vi "Set Aout Limit.vi"(8 "error in (no error)":errorcluster, 9 "firmware revision":string(combo), 10 "aout limit":T2={"ALimUpC (10.5)"=10.5, "ALimUpL (10.5)"=10.0, "ALimLoC (-10.5)"=-10.0, "ALimLoL (-10.5)"=-10.0}, 11 "VISA resource name":refnum<visa-resource-name>) -> (0 "error out":errorcluster, 2 "bridge error":T1, 3 "VISA resource name out":refnum<visa-resource-name>)   [LabVIEW 2020, in "Andeen-Hagerling 2700A.lvlib"]
doc: "Sets the upper and lower protection limits, respectively, of\nthe capacitance and loss channel output voltages in volts.\nThese protection limits apply only to voltage levels produced\nby the deviation subsystem. They do not limit the output\nderived from internal bias voltage sources."
uses:
  Andeen-Hagerling 2700A.lvlib
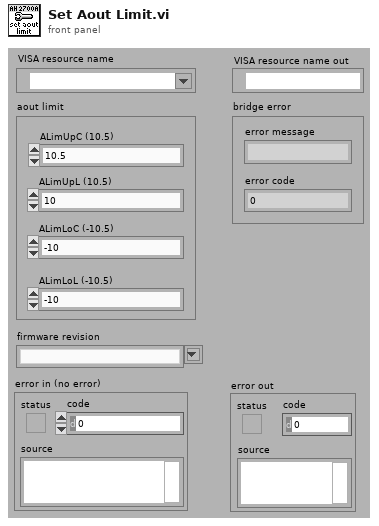
[diagram p1: front panel]
types:
  T1 = cluster{"error message":string, "error code":i32}
  T2 = cluster{"ALimUpC (10.5)":dbl, "ALimUpL (10.5)":dbl, "ALimLoC (-10.5)":dbl, "ALimLoL (-10.5)":dbl}
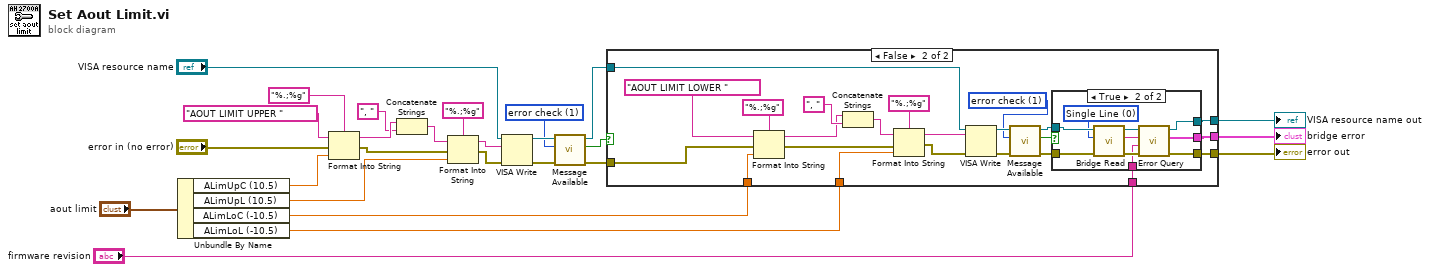
[diagram p0: block diagram]
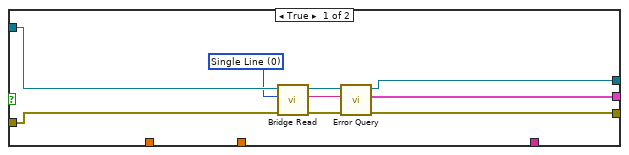
[diagram p2: hidden frame]
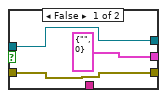
[diagram p3: hidden frame]
diagram:
  w1 = u16 1 items=["none", "error check", "multiline read", "infinite"] ("delay")
  n1 = Unbundle By Name("aout limit") -> ("ALimUpC (10.5)"=w17:dbl, "ALimUpL (10.5)"=w16:dbl, "ALimLoC (-10.5)"=w11:dbl, "ALimLoL (-10.5)"=w10:dbl)
  n2 = Format Into String(format string="%.;%g", initial string="AOUT LIMIT UPPER " ("command"), error in="error in (no error)", w17) -> (resulting string=w24:string, error out=w25:errorcluster)
  n3 = Concatenate Strings(w24, ", " ("command")) -> (w20:string)
  n4 = Format Into String(format string="%.;%g", initial string=w20, error in=w25, w16) -> (resulting string=w15:string, error out=w14:errorcluster)
  n5 = VISA Write(VISA resource name="VISA resource name", write buffer=w15, error in (no error)=w14) -> (VISA resource name out=w13:refnum<visa-resource-name>, error out=w12:errorcluster)  [unwired: 1 out]
  n6 = call "Message Available.vi"("error in (no error)"=w12, "delay"=w1, "VISA resource name"=w13) -> ("error out"=w3:errorcluster, "message available"=w2:bool, "VISA resource name out"=w4:refnum<visa-resource-name>)  [unwired: 6 in]
  n7 = case shown="False" w2 {
    tunnel: w11 -> [_ w44]
    tunnel: w10 -> [_ w43]
    tunnel: w4 -> [w31 w42]
    tunnel: "firmware revision" -> [_ w41]
    tunnel: [w30 w40] -> w8
    tunnel: [w29 w39] -> w7
    tunnel: [w28 w38] -> w6
    tunnel: w3 -> [w32 w37]
    frame True {
      w27 = u16 0 items=["Single Line", "Multi-Line"] ("Multiline")
      n8 = call "Bridge Read.vi"("error in (no error)"=w32, "multiline"=w27, "VISA resource name"=w31) -> ("error out"=w34:errorcluster, "read buffer"=w35:string, "VISA resource name out"=w33:refnum<visa-resource-name>)  [unwired: 6 in]
      n9 = call "Error Query.vi"("error in (no error)"=w34, "measurement line"=w35, "VISA resource name"=w33) -> ("error out"=w28:errorcluster, "bridge error"=w29:T1, "VISA resource name out"=w30:refnum<visa-resource-name>)  [unwired: 6 in]
    }
    frame False {
      w36 = u16 1 items=["none", "error check", "multiline read", "infinite"] ("delay")
      n10 = Format Into String(format string="%.;%g", initial string="AOUT LIMIT LOWER " ("command"), error in=w37, w44) -> (resulting string=w54:string, error out=w53:errorcluster)
      n11 = Concatenate Strings(w54, ", " ("command")) -> (w56:string)
      n12 = Format Into String(format string="%.;%g", initial string=w56, error in=w53, w43) -> (resulting string=w51:string, error out=w52:errorcluster)
      n13 = VISA Write(VISA resource name=w42, write buffer=w51, error in (no error)=w52) -> (VISA resource name out=w47:refnum<visa-resource-name>, error out=w46:errorcluster)  [unwired: 1 out]
      n14 = call "Message Available.vi"("error in (no error)"=w46, "delay"=w36, "VISA resource name"=w47) -> ("error out"=w48:errorcluster, "message available"=w50:bool, "VISA resource name out"=w49:refnum<visa-resource-name>)  [unwired: 6 in]
      n15 = case shown="True" w50 {
        tunnel: w49 -> [w60 w68]
        tunnel: w48 -> [w61 w67]
        tunnel: w41 -> [_ w66]
        tunnel: [w61 w65] -> w38
        tunnel: [w60 w64] -> w40
        tunnel: [T1 {"error message"="", "error code"=0} ("bridge error") w63] -> w39
        frame False {
        }
        frame True {
          w62 = u16 0 items=["Single Line", "Multi-Line"] ("Multiline")
          n16 = call "Bridge Read.vi"("error in (no error)"=w67, "multiline"=w62, "VISA resource name"=w68) -> ("error out"=w70:errorcluster, "read buffer"=w71:string, "VISA resource name out"=w69:refnum<visa-resource-name>)  [unwired: 6 in]
          n17 = call "Error Query.vi"("error in (no error)"=w70, "firmware revision"=w66, "measurement line"=w71, "VISA resource name"=w69) -> ("error out"=w65:errorcluster, "bridge error"=w63:T1, "VISA resource name out"=w64:refnum<visa-resource-name>)  [unwired: 5 in]
        }
      }
    }
  }
  "VISA resource name out" <- w8
  "error out" <- w6
  "bridge error" <- w7
